vi "角度to弧度-子.vi"(1 "角度":dbl) -> (0 "弧度":dbl)   [LabVIEW 2015]
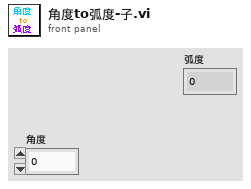
[diagram p1: front panel]
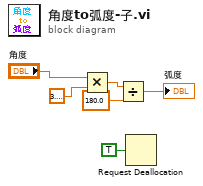
[diagram p0: block diagram]
diagram:
  n1 = Multiply(x="角度", y=3.141592653589793) -> (x*y=w4:dbl)
  n2 = Divide(x=w4, y=180.0) -> (x/y=→"弧度":dbl)
  n3 = Request Deallocation(TRUE ("标志")) -> ()
